vi "Measure.vi"(8 "error in (no error)":errorcluster, 11 "VISA resource name":refnum<visa-resource-name>) -> (0 "error out":errorcluster, 2 "Measured Value":dbl, 3 "VISA resource name out":refnum<visa-resource-name>)   [LabVIEW 2023, in "Keysight-34450A.lvlib"]
doc: "<b>Author:</b> Your NAME\n<b>Description:</b> >>>> Replace Me >>>"
uses:
  Keysight-34450A.lvlib
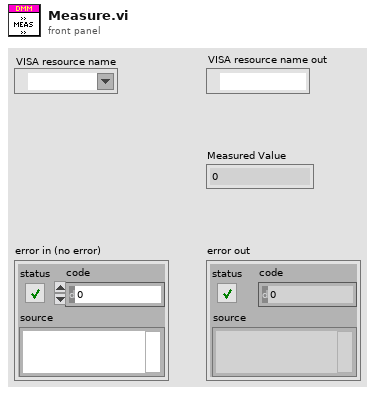
[diagram p1: front panel]
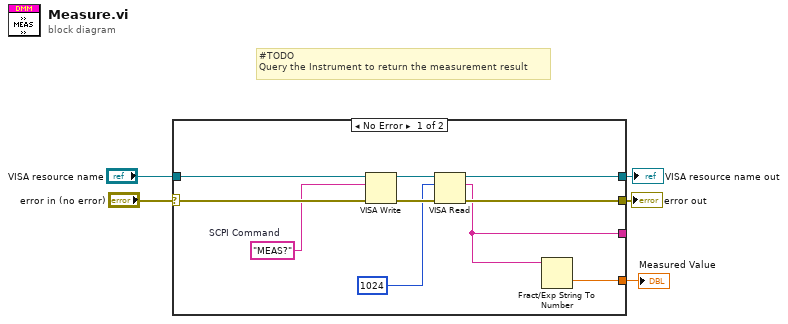
[diagram p0: block diagram]
diagram:
  # "#TODO\nQuery the Instrument to return the measurement result"
  n1 = case shown="No Error" "error in (no error)" {
    selector: "error in (no error)" -> [w9 w17]
    tunnel: [w15 w16] -> w5
    tunnel: [w13 w17] -> w3
    tunnel: "VISA resource name" -> [w10 w16]
    tunnel: [w7 _] -> _
    tunnel: [w6 _] -> w1
    frame No Error {
      w8 = "MEAS?"  # SCPI Command
      n2 = VISA Write(VISA resource name=w10, write buffer=w8, error in (no error)=w9) -> (VISA resource name out=w12:refnum<visa-resource-name>, error out=w14:errorcluster)  [unwired: 1 out]
      n3 = VISA Read(VISA resource name=w12, byte count=u32 1024, error in (no error)=w14) -> (VISA resource name out=w15:refnum<visa-resource-name>, read buffer=w7:string, error out=w13:errorcluster)  [unwired: 1 out]
      n4 = Fract/Exp String To Number(string=w7) -> (number=w6:dbl)  [unwired: 3 in, 1 out]
    }
    frame Error {
    }
  }
  "VISA resource name out" <- w5
  "error out" <- w3
  "Measured Value" <- w1
